vi "Get Teams.vi"(8 "error in (no error)":errorcluster, 11 "Asana in":refnum<class "Asana.lvclass">) -> (0 "error out":errorcluster, 2 "Teams out":T1(array[cluster]), 3 "Asana out":refnum<class "Asana.lvclass">)   [LabVIEW 2016, in "Asana.lvclass"]
uses:
  Asana.lvclass
  Asana.lvclass/Asana.ctl
  <vilib>/addons/_JKI.lib/REST Client/classes/REST Client/REST Client.lvclass
  <vilib>/addons/_JKI.lib/Serialization/JSON/JKI JSON Serialization.lvlib
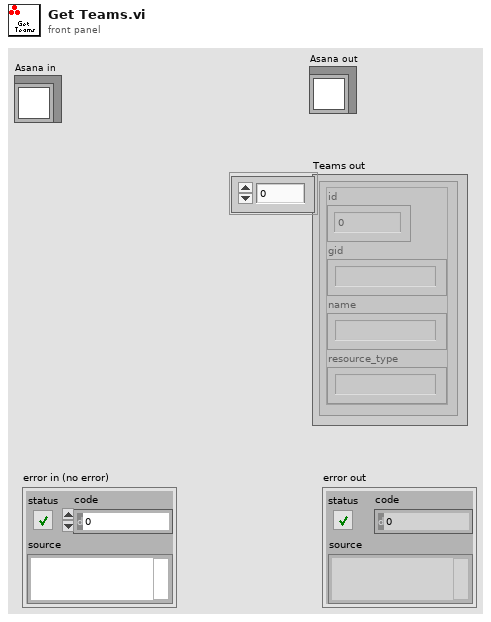
[diagram p1: front panel]
types:
  T1 = cluster{"id":i32, "gid":string, "name":string, "resource_type":string}[]
  T2 = cluster{"data":cluster{"id":i32, "gid":string, "name":string, "resource_type":string}[]}
  T3 = typedef "REST Client.lvlib/REST Client.lvclass/HTTP Header.ctl" = cluster{"header":string, "value":string}
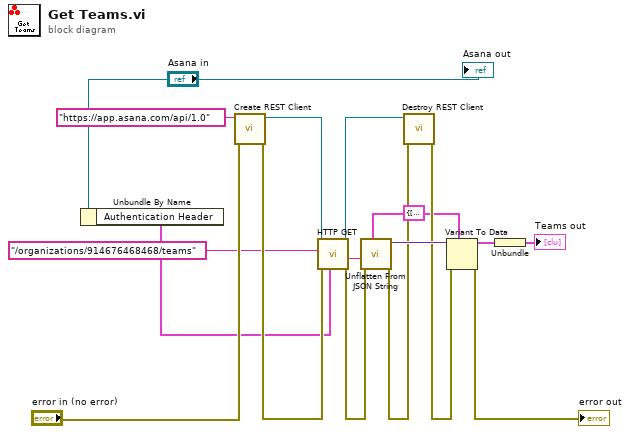
[diagram p0: block diagram]
diagram:
  w6 = T2 {"data"=[{"id"=11111111, "gid"="", "name"="", "resource_type"=""}, {"id"=-3, "gid"="", "name"="", "resource_type"=""}]}
  n1 = Unbundle By Name("Asana in") -> ("Authentication Header"=w1:T3[])
  n2 = call <vilib>:"Create REST Client.vi"("error in (no error)"="error in (no error)", "Base URL"="https://app.asana.com/api/1.0") -> ("error out"=w13:errorcluster, "REST Client out"=w16:refnum<class "REST Client.lvclass">)  [unwired: 8 in]
  n3 = call-dynamic "HTTP GET.vi"("request specific headers"=w1, "error in (no error)"=w13, "Path"="/organizations/914676468468/teams", "REST Client in"=w16) -> ("error out"=w10:errorcluster, "Response body"=w11:string, "REST Client out"=w15:refnum<class "REST Client.lvclass">)  [unwired: 2 in, 3 out]
  n4 = call <vilib>:"Unflatten From JSON String.vi"("Type and Defaults"=w6, "error in (no error)"=w10, "JSON String"=w11) -> ("error out"=w9:errorcluster, "Variant"=w12:variant)  [unwired: 7 in]
  n5 = call-dynamic "Destroy REST Client.vi"("error in (no error)"=w9, "REST Client in"=w15) -> ("error out"=w8:errorcluster)  [unwired: 9 in]
  n6 = Variant To Data(error in=w8, type=w6, Variant=w12) -> (data=w5:T2, error out=→"error out":errorcluster)
  n7 = Unbundle(w5) -> ("data"=→"Teams out":T1)
  "Asana out" <- "Asana in"
